vi "LJstreamM prepare custom formula.vi"(4 "Input Values":dbl[][](array[numeric]) format="%.2f", 6 "Variables Input":string[](array[string])=["v1", "v2", "v3", "v4"], 7 "NumFormulas":i32, 8 "error in (no error)":errorcluster, 10 "formulas":string[](array[string]), 11 "Input Formula":string) -> (0 "error out":errorcluster, 2 "Computed Values":dbl[][](array[numeric]), 3 "Output Formula":string)   [LabVIEW 2025]
doc: "Similar to the Formula Node function, but with variables that can be entered on the front panel."
uses:
  <vilib>/gmath/NI_Gmath.lvlib
panel:
  in  "Variables Output":string[](array[string])=["y"]
  # "Input = v\nOutput = y"
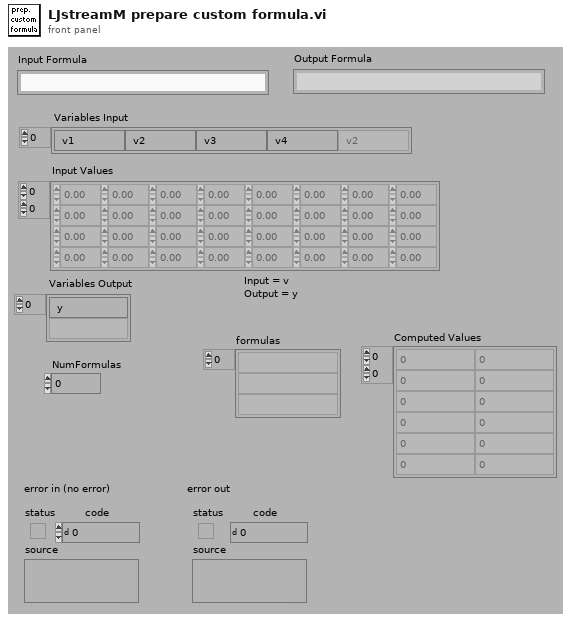
[diagram p1: front panel]
types:
  T1 = cluster{"Y Values":dbl[][], "Tables":i32[][][], "Variables input decode":i32[], "Variables output decode":i32[]}
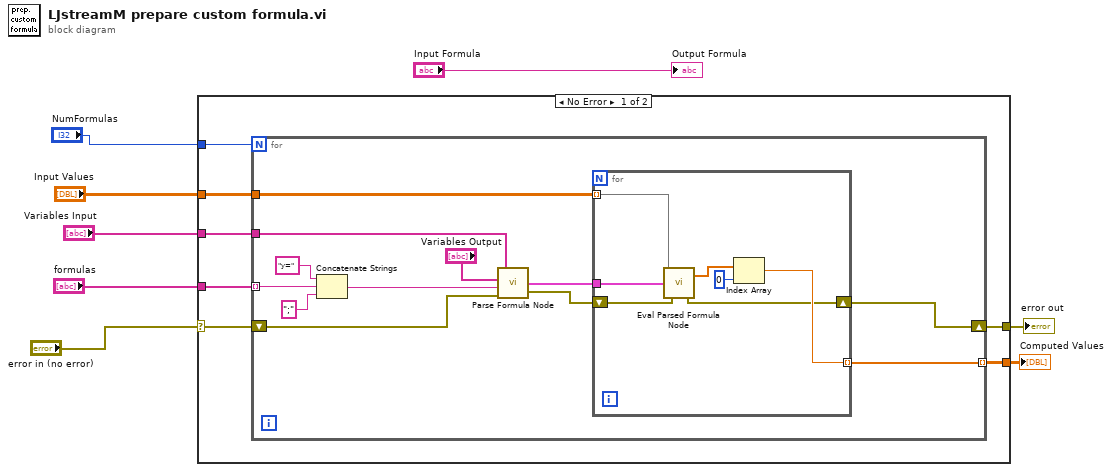
[diagram p0: block diagram]
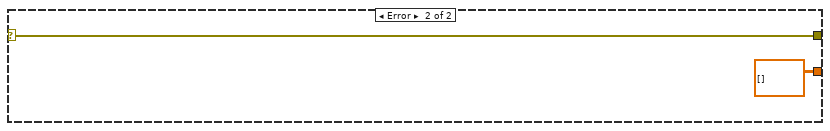
[diagram p2: hidden frame]
diagram:
  n1 = case shown="No Error" "error in (no error)" {
    selector: "error in (no error)" -> [w9 w35]
    tunnel: "Variables Input" -> [w15 _]
    tunnel: "Input Values" -> [w14 _]
    tunnel: "formulas" -> [w13 _]
    tunnel: "NumFormulas" -> [w12 _]
    tunnel: [w11 w35] -> w4
    tunnel: [w10 dbl[][] []] -> w2
    frame No Error {
      n2 = for {
        N: w12 -> [_]
        tunnel: w15 -> [w24]
        tunnel: w14 -> [w23]
        tunnel: w13 -> [w19] mode=indexing
        shift-right: [w17] -> w11
        shift-left: w9 -> [w18]
        tunnel: [w16] -> w10 mode=indexing
        n3 = Concatenate Strings("y=" ("Substring"), w19, ";" ("Substring")) -> (w20:string)
        n4 = call <vilib>:"Parse Formula Node.vi"("error in (no error)"=w18, "formula"=w20, "Variables Output"="Variables Output", "Variables Input"=w24) -> ("error out"=w27:errorcluster, "Parsed Formula Node"=w26:T1)
        n5 = for {
          tunnel: w23 -> [w28] mode=indexing
          tunnel: w26 -> [w34]
          tunnel: [w31] -> w16 mode=indexing
          shift-right: [w29] -> w17
          shift-left: w27 -> [w30]
          n6 = call <vilib>:"Eval Parsed Formula Node.vi"("error in (no error)"=w30, "Parsed Formula Node"=w34, "Input Values"=w28) -> ("error out"=w29:errorcluster, "Output Values"=w33:dbl[])
          n7 = Index Array(array=w33, index=0 ("Index")) -> (element=w31:dbl)
        }
      }
    }
    frame Error {
    }
  }
  "error out" <- w4
  "Computed Values" <- w2
  "Output Formula" <- "Input Formula"
